vi "Write Digital Output.vi"(7 "Device":string, 8 "error in":errorcluster, 9 "Line grouping":T1(ring), 10 "data":bool, 11 "Port_Line":string="Dev1/port0/line0") -> (0 "error out":errorcluster)   [LabVIEW 2015]
uses:
  <vilib>/DAQmx/write.llb/DAQmx Write (Digital Bool 1Line 1Point).vi
  <vilib>/DAQmx/create/channels.llb/DAQmx Create Channel (DO-Digital Output).vi
  <vilib>/DAQmx/miscellaneous.llb/DAQmx Fill In Error Info.vi
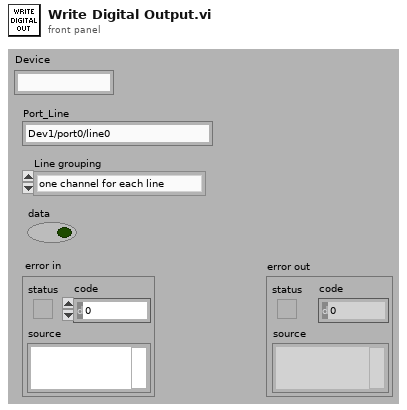
[diagram p1: front panel]
types:
  T1 = enum16{"one channel for each line", "one channel for all lines"}
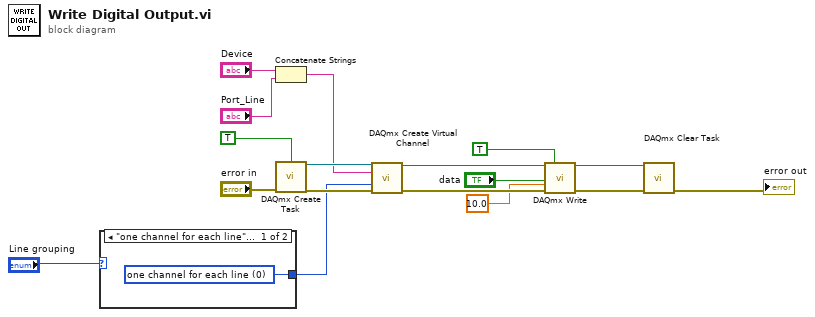
[diagram p0: block diagram]
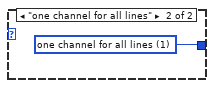
[diagram p2: hidden frame]
diagram:
  n1 = case shown="\"one channel for each line\", Default" "Line grouping" {
    tunnel: [w18 w19] -> w5
    frame "one channel for each line", Default {
      w18 = 0 items=["one channel for each line", "one channel for all lines"] ("line grouping")
    }
    frame "one channel for all lines" {
      w19 = 1 items=["one channel for each line", "one channel for all lines"] ("line grouping")
    }
  }
  n2 = Concatenate Strings("Device", "Port_Line") -> (w1:string)
  n3 = call <vilib>:"DAQmx Create Task.vi"("auto cleanup"=TRUE, "error in"="error in") -> ("task out"=w14:refnum<k21>, "error out"=w15:errorcluster)  [unwired: 12 in]
  n4 = call-poly <vilib>:"DAQmx Create Virtual Channel.vi"("task in"=w14, "lines"=w1, "line grouping"=w5, "error in"=w15) -> ("task out"=w13:refnum<k21>, "error out"=w12:errorcluster)  [unwired: 10 in]
  n5 = call-poly <vilib>:"DAQmx Write.vi"("task/channels in"=w13, "auto start"=TRUE, "data"="data", "timeout"=10.0, "error in"=w12) -> ("task out"=w8:refnum<k21>, "error out"=w9:errorcluster)  [unwired: 8 in, 1 out]
  n6 = call <vilib>:"DAQmx Clear Task.vi"("task in"=w8, "error in"=w9) -> ("error out"=→"error out":errorcluster)  [unwired: 13 in]
